vi "Query Marker.vi"(8 "error in (no error)":errorcluster, 10 "Marker Number":u8=1, 11 "VNA-FieldFox in":refnum<class "VNA-FieldFox.lvclass">) -> (0 "error out":errorcluster, 1 "Data":dbl, 2 "Frequency":dbl, 3 "VNA-FieldFox out":refnum<class "VNA-FieldFox.lvclass">)   [LabVIEW 2020, in "VNA-FieldFox.lvclass"]
doc: "Query the marker on the active trace"
uses:
  VNA-FieldFox.lvclass
  Vector Network Analyzer.lvclass
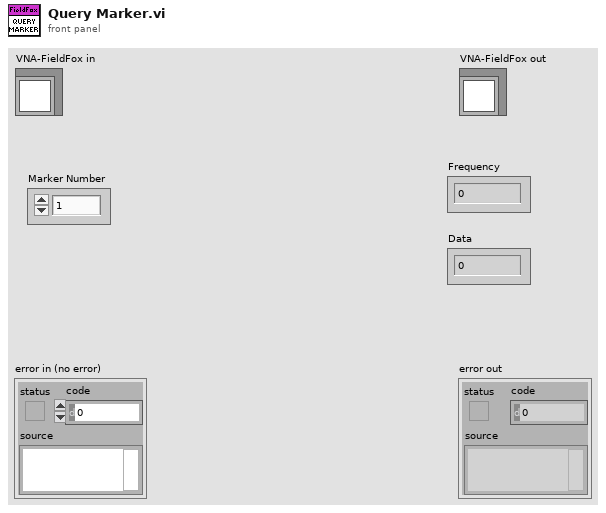
[diagram p1: front panel]
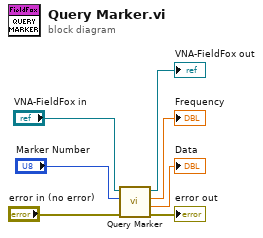
[diagram p0: block diagram]
diagram:
  n1 = call-parent "Query Marker.vi"("error in (no error)"="error in (no error)", "Marker Number"="Marker Number", "Vector Network Analyzer in"="VNA-FieldFox in") -> ("error out"=→"error out":errorcluster, "Data"=→"Data":dbl, "Frequency"=→"Frequency":dbl, "Vector Network Analyzer out"=→"VNA-FieldFox out":refnum<class "VNA-FieldFox.lvclass">)  [unwired: 5 in]
